vi "NXT_MIDBRAIN Compare First Charachter.vi"(4 "string":string, 5 "ModuleName":string, 6 "error in (no error)":errorcluster, 7 "Refnum in":T1) -> (1 "Boolean":bool, 2 "error out":errorcluster, 3 "Refnum Out":T1)   [LabVIEW 2012]
uses:
  <vilib>/NXT/NXT Controls/NXTSyscallRefnum.ctl
  <resource>/objmgr/NXTInputOutput.rc
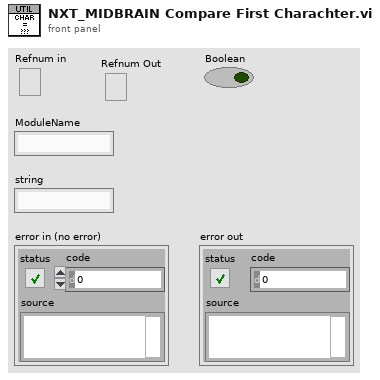
[diagram p1: front panel]
types:
  T1 = typedef "NXTSyscallRefnum.ctl" = refnum<k21>
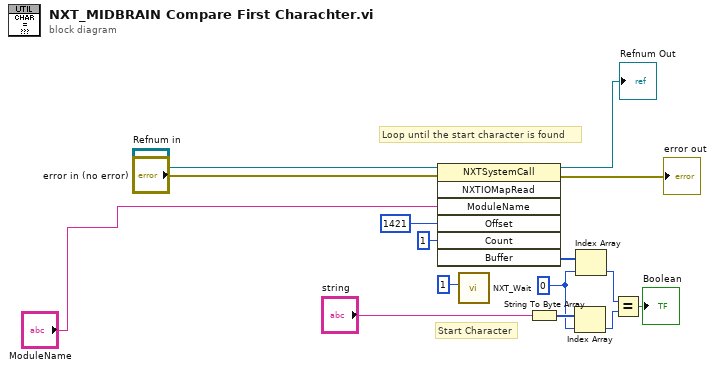
[diagram p0: block diagram]
diagram:
  w8 = 0 ("index")
  # "Loop until the start character is found"
  # "Start Character"
  n1 = invoke class="NXTSystemCall" method="NXTIOMapRead"(reference="Refnum in", error in="error in (no error)", "ModuleName"="ModuleName", "Offset"=1421, "Count"=u16 1) -> (reference out=→"Refnum Out":T1, error out=→"error out":errorcluster, "Buffer"=w6:u8[])  [unwired: 2 in, 4 out]
  n2 = call <vilib>:"NXT_Wait.vi"("Wait (ms)"=u32 1) -> ()  [unwired: 9 in, 2 out]
  n3 = String To Byte Array(string="string") -> (unsigned byte array=w9:u8[])
  n4 = Index Array(array=w9, index=w8) -> (element=w11:u8)
  n5 = Index Array(array=w6, index=w8) -> (element=w7:u8)
  n6 = Equal?(x=w7, y=w11) -> (x = y?=→"Boolean":bool)
